vi "Initialize.vi"(8 "error in (no error)":errorcluster, 11 "PacificPowerSource in":refnum<class "PacificPowerSource.lvclass">) -> (0 "error out":errorcluster, 3 "PacificPowerSource out":refnum<class "PacificPowerSource.lvclass">)   [LabVIEW 2018, in "AcPwrPlugins.lvlib" / "PacificPowerSource.lvclass"]
doc: "This VI establishes communication to the instrument and optionally performs an instrument identification query and/or an instrument reset. It also places the instrument in a default state needed for other instrument driver operations. Therefore, call this VI before calling other instrument driver VIs for this instrument. Generally, you need to call the Initialize VI only once at the beginning of an application.\n\n<b>Note:</b>\nYou can clear device while you enable \"Clear Device\", and the AC power will restart."
uses:
  PacificPowerSource.lvclass
  <instrlib>/Pacific Power UPC Series/Pacific Power UPC Series.lvlib
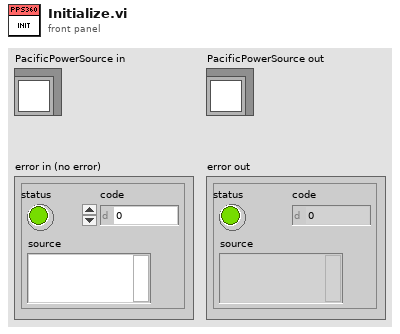
[diagram p1: front panel]
types:
  T1 = cluster{"Boolean":bool, "VISA Resource name":refnum<visa-resource-name>}[]
  T2 = typedef "AcPwrPlugins.lvlib/PacificPowerSource.lvclass/DeviceSettings.ctl" = cluster{"Handle":string, "Connected":bool, "Clear Device (F)":bool, "btnIdQuery":bool, "btnReset":bool, "Program #":cluster{"Phase B (Degrees)":i32, "Waveform A (1: Sine)":i32, "Voltage Level (Va)":dbl, "Program Number (0)":i32, "Voltage Level (Vb) ":dbl, "Form (3: Three)":u16, "Coupling  (0: Direct)":u16, "Frequency (45Hz)":dbl, "Current Limit (40A)":dbl, "Phase C (Degrees)":i32, "Voltage Level (Vc)":dbl, "Waveform B (1: Sine)":i32, "Waveform C (1: Sine)":i32}[], "Impedance Parameters (off, 0.00)":cluster{"State":bool, "Impedance":dbl}, "Transient Execution (F)":bool, "OutputEnabled":bool, "Source Range":cluster{"Frequency Minimum (45 Hz)":dbl, "Frequency Maximum (1200 Hz)":dbl, "Voltage Maximum (V)":dbl, "Voltage Minimum (V)":dbl, "Range Control (0: Auto)":u16, "Initial Voltage (0V)":u16, "Frequency Range (600Hz)":u16}, "Port Type":enum16{"GPIB", "Serial"}}[]
  T3 = cluster{"Handle":string, "Connected":bool, "Clear Device (F)":bool, "btnIdQuery":bool, "btnReset":bool, "Program #":cluster{"Phase B (Degrees)":i32, "Waveform A (1: Sine)":i32, "Voltage Level (Va)":dbl, "Program Number (0)":i32, "Voltage Level (Vb) ":dbl, "Form (3: Three)":u16, "Coupling  (0: Direct)":u16, "Frequency (45Hz)":dbl, "Current Limit (40A)":dbl, "Phase C (Degrees)":i32, "Voltage Level (Vc)":dbl, "Waveform B (1: Sine)":i32, "Waveform C (1: Sine)":i32}[], "Impedance Parameters (off, 0.00)":cluster{"State":bool, "Impedance":dbl}, "Transient Execution (F)":bool, "OutputEnabled":bool, "Source Range":cluster{"Frequency Minimum (45 Hz)":dbl, "Frequency Maximum (1200 Hz)":dbl, "Voltage Maximum (V)":dbl, "Voltage Minimum (V)":dbl, "Range Control (0: Auto)":u16, "Initial Voltage (0V)":u16, "Frequency Range (600Hz)":u16}, "Port Type":enum16{"GPIB", "Serial"}}
  T4 = cluster{"Handle Connected?":bool, "VISA Resource name":refnum<visa-resource-name>}
  T5 = cluster{"Handle Connected?":bool, "VISA Resource name":refnum<visa-resource-name>}[]
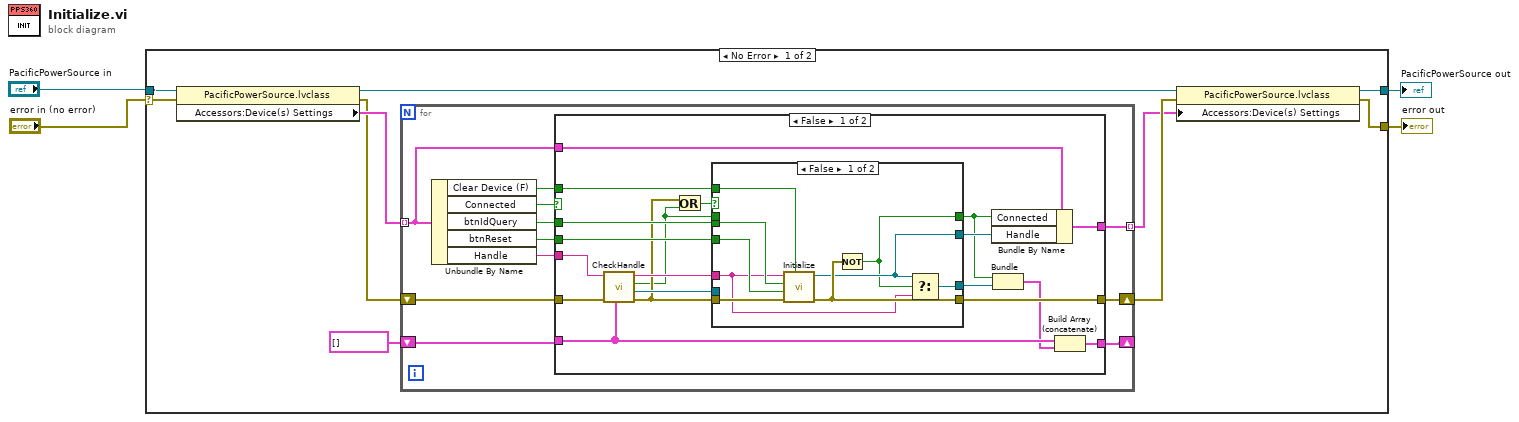
[diagram p0: block diagram]
diagram:
  n1 = case shown="No Error" "error in (no error)" {
    selector: "error in (no error)" -> [w11 w60]
    tunnel: "PacificPowerSource in" -> [w14 w61]
    tunnel: [w8 w61] -> w2
    tunnel: [w7 w60] -> w1
    frame No Error {
      n2 = property class="PacificPowerSource.lvclass"(reference=w14, error in=w11) -> (reference out=w12:refnum<class "PacificPowerSource.lvclass">, error out=w10:errorcluster, "Accessors:Device(s) Settings"=w13:T2)
      n3 = for {
        shift-right: [w24] -> w9
        shift-left: w10 -> [w25]
        tunnel: w13 -> [w23] mode=indexing
        tunnel: [w22] -> w6 mode=indexing
        shift-right: [w15] -> _
        shift-left: T1 [] ("Array") -> [w16]
        n4 = Unbundle By Name(w23) -> ("Clear Device (F)"=w20:bool, "Connected"=w21:bool, "btnIdQuery"=w19:bool, "btnReset"=w18:bool, "Handle"=w17:string)
        n5 = case shown="False" w21 {
          tunnel: w25 -> [w38 w59]
          tunnel: [w40 w59] -> w24
          tunnel: w18 -> [w42 _]
          tunnel: w19 -> [w41 _]
          tunnel: w23 -> [w29 w58]
          tunnel: [w44 w58] -> w22
          tunnel: w20 -> [w39 _]
          tunnel: w17 -> [w37 _]
          tunnel: w16 -> [w31 w57]
          tunnel: [w30 w57] -> w15
          frame False {
            n6 = call "CheckHandle.vi"("Array"=w31, "Error In"=w38, "Handle In"=w37) -> ("Error Out"=w33:errorcluster, "VISA Resource name"=w34:refnum<visa-resource-name>, "Handle Connected?"=w32:bool, "Handle Out"=w36:string)  [unwired: 5 in]
            n7 = Or(x=w33, y=w32) -> (x .or. y?=w35:bool)
            n8 = case shown="False" w35 {
              tunnel: [w46 w55] -> w27
              tunnel: w33 -> [w53 w56]
              tunnel: [w48 w54] -> w43
              tunnel: w42 -> [w52 _]
              tunnel: w41 -> [w51 _]
              tunnel: [w50 w56] -> w40
              tunnel: w39 -> [w49 _]
              tunnel: w36 -> [w47 _]
              tunnel: w34 -> [_ w54]
              tunnel: w32 -> [_ w55]
              tunnel: [w45 w54] -> w28
              frame False {
                n9 = call <instrlib>:"Initialize.vi"("Clear Device (False)"=w49, "error in (no error)"=w53, "Reset (True)"=w52, "ID Query (True)"=w51, "VISA resource name"=w47) -> ("error out"=w50:errorcluster, "VISA resource name out"=w48:refnum<visa-resource-name>)  [unwired: 5 in]
                n10 = Not(x=w50) -> (.not. x?=w46:bool)
                n11 = Select(t=w48, s=w46, f=w47) -> (s? t:f=w45:refnum<visa-resource-name>)
              }
              frame True {
              }
            }
            n12 = Bundle By Name(cluster=w29, "Connected"=w27, "Handle"=w43) -> (w44:T3)
            n13 = Bundle("Handle Connected?"=w27, "VISA Resource name"=w28) -> (w26:T4)  [unwired: 1 in]
            n14 = Build Array (concatenate)(w31, w26) -> (w30:T5)
          }
          frame True {
          }
        }
      }
      n15 = property class="PacificPowerSource.lvclass"(reference=w12, error in=w9, "Accessors:Device(s) Settings"=w6) -> (reference out=w8:refnum<class "PacificPowerSource.lvclass">, error out=w7:errorcluster)
    }
    frame Error {
    }
  }
  "error out" <- w1
  "PacificPowerSource out" <- w2
